vi "Idle_InterpretCommand.vi"(8 "error in":errorcluster, 11 "Input Command":string="MCS_NCAR_Setup") -> (0 "error out":errorcluster, 3 "What to Do":string="Initial setup of NCAR MCS")   [LabVIEW 2012]
uses:
  GlobalVariables_DIALMain.vi
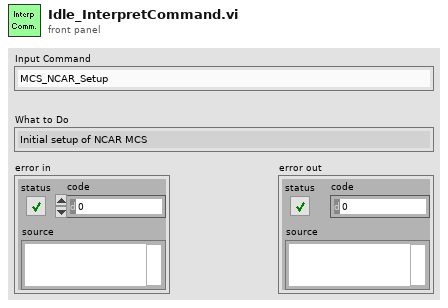
[diagram p1: front panel]
types:
  T1 = enum32{"Invalid", "Standard", "Closed", "Hidden", "Minimized", "Maximized"}
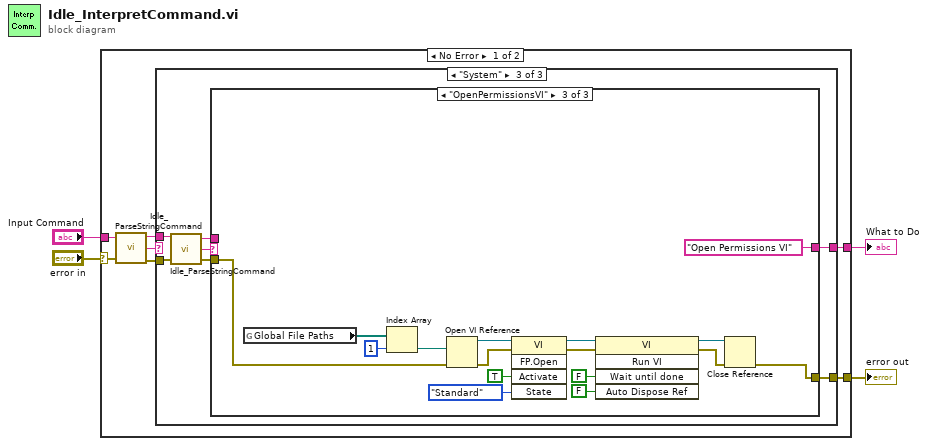
[diagram p0: block diagram]
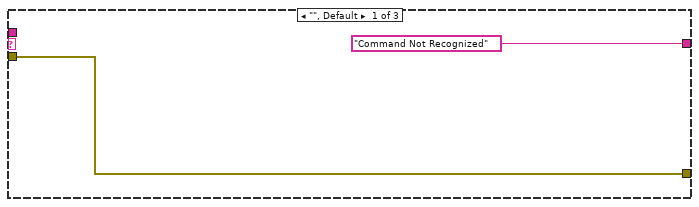
[diagram p2: hidden frame]
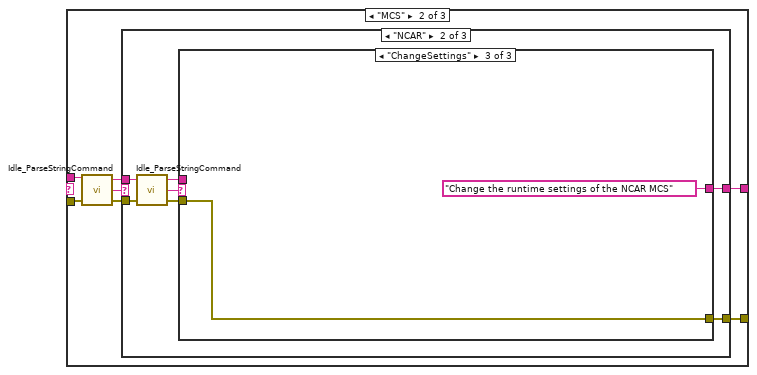
[diagram p3: hidden frame]
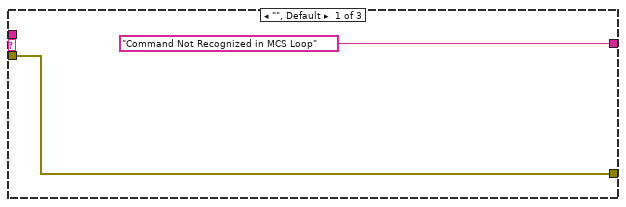
[diagram p4: hidden frame]
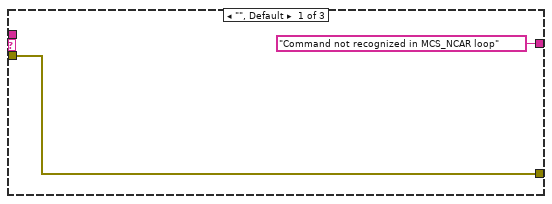
[diagram p5: hidden frame]
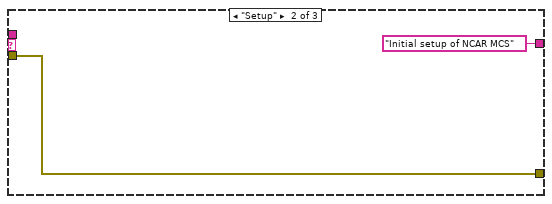
[diagram p6: hidden frame]
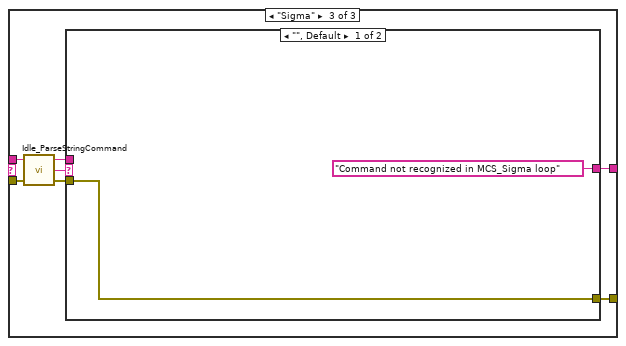
[diagram p7: hidden frame]
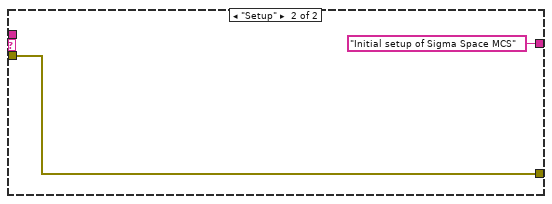
[diagram p8: hidden frame]
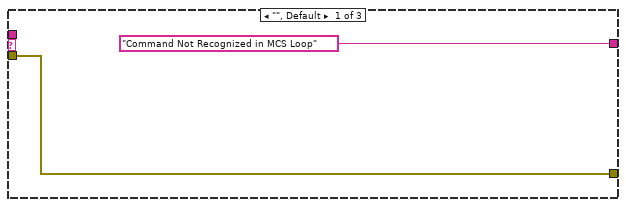
[diagram p9: hidden frame]
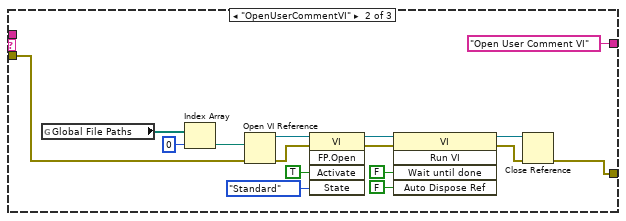
[diagram p10: hidden frame]
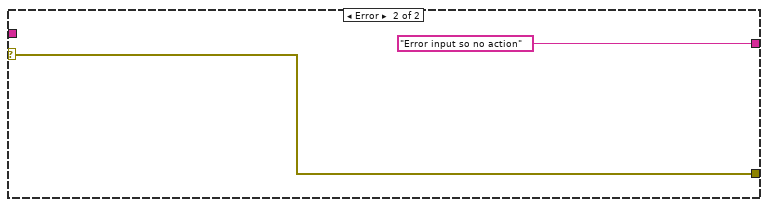
[diagram p11: hidden frame]
diagram:
  n1 = case shown="No Error" "error in" {
    selector: "error in" -> [w5 w88]
    tunnel: "Input Command" -> [w11 _]
    tunnel: [w7 "Error input so no action"] -> w3
    tunnel: [w6 w88] -> w2
    frame No Error {
      n2 = call "Idle_ParseStringCommand.vi"("error in"=w5, "Input Command"=w11) -> ("error out"=w8:errorcluster, "Command"=w9:string, "Remaining String"=w10:string)  [unwired: 1 in]
      n3 = case shown="\"System\"" w9 {
        tunnel: w10 -> [_ w20 w53]
        tunnel: w8 -> [w12 w19 w52]
        tunnel: ["Command Not Recognized" w15 w48] -> w7
        tunnel: [w12 w14 w47] -> w6
        frame "", Default {
        }
        frame "MCS" {
          n4 = call "Idle_ParseStringCommand.vi"("error in"=w19, "Input Command"=w20) -> ("error out"=w16:errorcluster, "Command"=w17:string, "Remaining String"=w18:string)  [unwired: 1 in]
          n5 = case shown="\"NCAR\"" w17 {
            tunnel: w18 -> [_ w28 w41]
            tunnel: w16 -> [w21 w27 w40]
            tunnel: ["Command Not Recognized in MCS Loop" w29 w42] -> w15
            tunnel: [w21 w23 w36] -> w14
            frame "", Default {
            }
            frame "NCAR" {
              n6 = call "Idle_ParseStringCommand.vi"("error in"=w27, "Input Command"=w28) -> ("error out"=w25:errorcluster, "Command"=w26:string, "Remaining String"=w24:string)  [unwired: 1 in]
              n7 = case shown="\"ChangeSettings\"" w26 {
                tunnel: ["Command not recognized in MCS_NCAR loop" "Initial setup of NCAR MCS" "Change the runtime settings of the NCAR MCS"] -> w29
                tunnel: w25 -> [w30 w32 w34]
                tunnel: w24 -> [_ _ _]
                tunnel: [w30 w32 w34] -> w23
                frame "", Default {
                }
                frame "Setup" {
                }
                frame "ChangeSettings" {
                }
              }
            }
            frame "Sigma" {
              n8 = call "Idle_ParseStringCommand.vi"("error in"=w40, "Input Command"=w41) -> ("error out"=w38:errorcluster, "Command"=w39:string, "Remaining String"=w37:string)  [unwired: 1 in]
              n9 = case shown="\"\", Default" w39 {
                tunnel: ["Command not recognized in MCS_Sigma loop" "Initial setup of Sigma Space MCS"] -> w42
                tunnel: w38 -> [w43 w45]
                tunnel: w37 -> [_ _]
                tunnel: [w43 w45] -> w36
                frame "", Default {
                }
                frame "Setup" {
                }
              }
            }
          }
        }
        frame "System" {
          n10 = call "Idle_ParseStringCommand.vi"("error in"=w52, "Input Command"=w53) -> ("error out"=w49:errorcluster, "Command"=w50:string, "Remaining String"=w51:string)  [unwired: 1 in]
          n11 = case shown="\"OpenPermissionsVI\"" w50 {
            tunnel: w51 -> [_ _ _]
            tunnel: w49 -> [w54 w70 w86]
            tunnel: ["Command Not Recognized in MCS Loop" "Open User Comment VI" "Open Permissions VI"] -> w48
            tunnel: [w54 w59 w75] -> w47
            frame "", Default {
            }
            frame "OpenUserCommentVI" {
              n12 = global read "GlobalVariables_DIALMain.vi" "Global File Paths"() -> (w71:path[])
              n13 = Index Array(array=w71, index=0) -> (element=w58:path)
              n14 = Open VI Reference(vi path=w58, error in (no error)=w70) -> (vi reference=w69:refnum<vi>, error out=w68:errorcluster)  [unwired: 4 in]
              n15 = invoke class="VI" method="FP.Open"(reference=w69, error in=w68, "Activate"=TRUE ("Wait Until Done"), "State"=T1."Standard") -> (reference out=w65:refnum<vi>, error out=w64:errorcluster)  [unwired: 1 in, 3 out]
              n16 = invoke class="VI" method="Run VI"(reference=w65, error in=w64, "Wait until done"=FALSE ("Wait Until Done"), "Auto Dispose Ref"=FALSE ("Auto Dispose Reference")) -> (reference out=w61:refnum<vi>, error out=w60:errorcluster)  [unwired: 1 in, 3 out]
              n17 = Close Reference(reference=w61, error in (no error)=w60) -> (error out=w59:errorcluster)
            }
            frame "OpenPermissionsVI" {
              n18 = global read "GlobalVariables_DIALMain.vi" "Global File Paths"() -> (w87:path[])
              n19 = Index Array(array=w87, index=1) -> (element=w74:path)
              n20 = Open VI Reference(vi path=w74, error in (no error)=w86) -> (vi reference=w85:refnum<vi>, error out=w84:errorcluster)  [unwired: 4 in]
              n21 = invoke class="VI" method="FP.Open"(reference=w85, error in=w84, "Activate"=TRUE ("Wait Until Done"), "State"=T1."Standard") -> (reference out=w81:refnum<vi>, error out=w80:errorcluster)  [unwired: 1 in, 3 out]
              n22 = invoke class="VI" method="Run VI"(reference=w81, error in=w80, "Wait until done"=FALSE ("Wait Until Done"), "Auto Dispose Ref"=FALSE ("Auto Dispose Reference")) -> (reference out=w77:refnum<vi>, error out=w76:errorcluster)  [unwired: 1 in, 3 out]
              n23 = Close Reference(reference=w77, error in (no error)=w76) -> (error out=w75:errorcluster)
            }
          }
        }
      }
    }
    frame Error {
    }
  }
  "What to Do" <- w3
  "error out" <- w2
